vi "S4GUI_002.vi"(7 "Tab ObsEng":enum32{"Obs", "CCD modes", "Eng"}(tab)) -> ()   [LabVIEW 2018] (continued)
            n1189 = call-dynamic "Read TelFocus.lvclass.vi"("error in (no error)"=w302, "S4GUI in"=w303) -> ("error out"=w300:errorcluster, "TelFocus.lvclass"=w301:refnum<class "TelFocus.lvclass">)  [unwired: 7 in, 1 out]
            n1190 = Select(t="STOP", s=w320, f="INIT") -> (s? t:f=w319:string)
            n1191 = call-dynamic "Read focus #stepsdone.vi"("error in (no error)"=w300, "TelFocus in"=w301) -> ("focus #stepsdone"=→"steps done":u32)  [unwired: 7 in, 2 out]
            n1192 = property on="Init mode" class="Bool"(error in=w302, "Blinking"=w320, "Caption.Visible"=w320, "BoolText.Text"=w319) -> (error out=w321:errorcluster)  [unwired: 1 in, 1 out]
            n1193 = call-dynamic "Read cyclesDone.vi"("error in (no error)"=w321, "S4GUI in"=w303) -> ("error out"=w313:errorcluster, "cyclesDone"=w305:u32, "S4GUI out"=w315:refnum<class "S4GUI.lvclass">)  [unwired: 7 in]
            "#Cycles Done" <- w305
            n1194 = call-dynamic "Read cycles wprot.vi"("error in (no error)"=w313, "S4GUI in"=w315) -> ("cycles wprot"=→"Cycles Counter":u32)  [unwired: 7 in, 2 out]
            n1195 = Number To Decimal String(number=w305) -> (decimal integer string=w306:string)  [unwired: 1 in]
            n1196 = Concatenate Strings("#Cycles Done ", w306) -> (w304:string)
            n1197 = property on="#Cycles Done" class="Slide (strict)"("Caption.Text"=w304) -> ()  [unwired: 2 in, 2 out]
            n1198 = call "Read Instrument.lvclass.vi"("error in (no error)"=w313, "S4ACS_GUI in"=w315) -> ("error out"=w330:errorcluster, "Instrument.lvclass"=w328:refnum<class "Instrument.lvclass">, "S4ACS_GUI out"=w331:refnum<class "S4GUI.lvclass">)  [unwired: 7 in]
            n1199 = call-dynamic "Write mode.vi"("error in (no error)"=w330, "mode"=w316, "Instrument in"=w328) -> ("error out"=w329:errorcluster, "Instrument out"=w327:refnum<class "Instrument.lvclass">)  [unwired: 7 in]
            n1200 = call "Write Instrument.lvclass.vi"("error in (no error)"=w329, "Instrument.lvclass"=w327, "S4ACS_GUI in"=w331) -> ("error out"=w311:errorcluster, "S4ACS_GUI out"=w312:refnum<class "S4GUI.lvclass">)  [unwired: 7 in]
            n1201 = call-dynamic "Read Error Msg.vi"("error in (no error)"=w311, "S4GUI in"=w312) -> ("error out"=w308:errorcluster, "Error Msg"=w290:string, "S4GUI out"=w295:refnum<class "S4GUI.lvclass">)  [unwired: 7 in]
            "Last Error" <- w290
            n1202 = Match Pattern(string=w290, regular expression=w309) -> (match substring=w310:string)  [unwired: 1 in, 3 out]
            n1203 = Equal?(x=w310, y=w309) -> (x = y?=w289:bool)
            n1204 = Match Pattern(string=w290, regular expression=w291) -> (match substring=w292:string)  [unwired: 1 in, 3 out]
            n1205 = Equal?(x=w292, y=w291) -> (x = y?=w288:bool)
            n1206 = Or(x=w289, y=w288) -> (x .or. y?=w287:bool)
            n1207 = property on="Last Error" class="Str"(error in=w308, "Blinking"=w287) -> (error out=w293:errorcluster)  [unwired: 1 in, 1 out]
            n1208 = call "Read Instrument.lvclass.vi"("error in (no error)"=w293, "S4ACS_GUI in"=w295) -> ("error out"=w297:errorcluster, "Instrument.lvclass"=w296:refnum<class "Instrument.lvclass">, "S4ACS_GUI out"=w285:refnum<class "S4GUI.lvclass">)  [unwired: 7 in]
            n1209 = call-dynamic "Read mode.vi"("error in (no error)"=w297, "Instrument in"=w296) -> ("error out"=w286:errorcluster, "mode"=w298:bool)  [unwired: 7 in, 1 out]
            n1210 = while {
              tunnel: w298 -> [w341]
              shift-right: [w337] -> _
              shift-left: _ -> [w340]
              shift-right: [w338] -> _
              shift-left: _ -> [w339]
              stop <- TRUE stop-if-true
              n1211 = case shown="False" w341 {
                tunnel: w340 -> [w343 w362]
                tunnel: [w344 w361] -> w337
                tunnel: w339 -> [w346 w360]
                tunnel: [w345 w359] -> w338
                frame True {
                  # "polarimetria"
                  n1212 = case shown="False" w346 {
                    selector: w346 -> [w356 w358]
                    tunnel: [w355 w358] -> w345
                    tunnel: [FALSE FALSE] -> w344
                    tunnel: w343 -> [_ _]
                    frame False {
                      w353 = 11
                      w350 = 80
                      w349 = 12900
                      # "Valor médio\ndo curso do foco."
                      n1213 = local write "Start focus"(w349) -> ()
                      n1214 = local write "Step focus"(w350) -> ()
                      n1215 = local write "#steps"(w353) -> ()
                      n1216 = Quotient & Remainder(x=w353, y=2) -> (floor(x/y)=w351:i32)  [unwired: 1 out]
                      n1217 = Multiply(x=w350, y=w351) -> (x*y=w348:i32)
                      n1218 = Add(x=w349, y=w348) -> (x+y=w347:i32)
                      n1219 = local write "Target focus 2"(w347) -> ()
                      n1220 = local write "Target focus"(w347) -> ()
                      n1221 = Not(x=w356) -> (.not. x?=w355:bool)
                    }
                    frame True {
                    }
                  }
                }
                frame False {
                  # "fotometria"
                  n1222 = case shown="False" w362 {
                    selector: w362 -> [w371 w374]
                    tunnel: [w370 w374] -> w361
                    tunnel: w360 -> [_ _]
                    tunnel: [FALSE FALSE] -> w359
                    frame False {
                      w366 = 11
                      w365 = 100
                      w364 = 13400
                      # "Valor médio\ndo curso do foco."
                      n1223 = local write "Start focus"(w364) -> ()
                      n1224 = local write "Step focus"(w365) -> ()
                      n1225 = local write "#steps"(w366) -> ()
                      n1226 = Quotient & Remainder(x=w366, y=2) -> (floor(x/y)=w368:i32)  [unwired: 1 out]
                      n1227 = Multiply(x=w365, y=w368) -> (x*y=w367:i32)
                      n1228 = Add(x=w364, y=w367) -> (x+y=w363:i32)
                      n1229 = local write "Target focus"(w363) -> ()
                      n1230 = local write "Target focus 2"(w363) -> ()
                      n1231 = Not(x=w371) -> (.not. x?=w370:bool)
                    }
                    frame True {
                    }
                  }
                }
              }
            }
            n1232 = call-dynamic "Read exit.vi"("error in (no error)"=w286, "S4GUI in"=w285) -> ("error out"=w284:errorcluster, "exit"=w283:bool, "S4GUI out"=w282:refnum<class "S4GUI.lvclass">)  [unwired: 7 in]
          }
        }
      }
      event "Lambda Selector": Mouse Down? {
        n1233 = event-data() -> ()  [unwired: 1 in, 7 out]
        n1234 = First Call?() -> (First Call?: T/F=w1982:bool)
        n1235 = case shown="True" w1982 {
          tunnel: w1984 -> [w1986 w1988]
          tunnel: [w1986 w1987] -> w1983
          frame False {
          }
          frame True {
            w1990 = u16 0 items=["OFF", "Lambda/2", "Lambda/4"] ("Lambda Selector")
            n1236 = property on="Lambda Selector" class="Ring (strict)"(error in=w1988, "Value"=w1990) -> (error out=w1991:errorcluster)  [unwired: 1 in, 1 out]
            n1237 = property on="Lambda Selector" class="Ring (strict)"(error in=w1991, "RingText.Text"="OFF" ("Boolean Text.Text")) -> (error out=w1987:errorcluster)  [unwired: 1 in, 1 out]
          }
        }
        n1238 = event-data() -> ()  [unwired: 2 in, 1 out]
      }
      event "object suffix": Key Down; "object suffix": Key Repeat {
        n1239 = event-data() -> ("Char"=w1992:i16)  [unwired: 1 in]
        "charKeyboardInteger" <- w1992
        n1240 = call-dynamic "Write charSuffix.vi"("error in (no error)"=w1995, "charSuffix"=w1992, "S4GUI in"=w1996) -> ("error out"=w1993:errorcluster, "S4GUI out"=w1994:refnum<class "S4GUI.lvclass">)  [unwired: 7 in]
      }
      event "dflat suffix": Key Down; "dflat suffix": Key Repeat {
        n1241 = event-data() -> ("Char"=w1999:i16)  [unwired: 1 in]
        n1242 = call-dynamic "Write charSuffix.vi"("error in (no error)"=w2000, "charSuffix"=w1999, "S4GUI in"=w2001) -> ("error out"=w1997:errorcluster, "S4GUI out"=w1998:refnum<class "S4GUI.lvclass">)  [unwired: 7 in]
      }
      event "sflat suffix": Key Down; "sflat suffix": Key Repeat {
        n1243 = event-data() -> ("Char"=w2004:i16)  [unwired: 1 in]
        n1244 = call-dynamic "Write charSuffix.vi"("error in (no error)"=w2005, "charSuffix"=w2004, "S4GUI in"=w2006) -> ("error out"=w2002:errorcluster, "S4GUI out"=w2003:refnum<class "S4GUI.lvclass">)  [unwired: 7 in]
      }
      event "dark suffix": Key Down; "dark suffix": Key Repeat {
        n1245 = event-data() -> ("Char"=w2009:i16)  [unwired: 1 in]
        n1246 = call-dynamic "Write charSuffix.vi"("error in (no error)"=w2010, "charSuffix"=w2009, "S4GUI in"=w2011) -> ("error out"=w2007:errorcluster, "S4GUI out"=w2008:refnum<class "S4GUI.lvclass">)  [unwired: 7 in]
      }
      event "zero suffix": Key Down; "zero suffix": Key Repeat {
        n1247 = event-data() -> ("Char"=w2014:i16)  [unwired: 1 in]
        n1248 = call-dynamic "Write charSuffix.vi"("error in (no error)"=w2015, "charSuffix"=w2014, "S4GUI in"=w2016) -> ("error out"=w2012:errorcluster, "S4GUI out"=w2013:refnum<class "S4GUI.lvclass">)  [unwired: 7 in]
      }
      event "focus suffix": Key Down; "focus suffix": Key Repeat {
        n1249 = event-data() -> ("Char"=w2019:i16)  [unwired: 1 in]
        n1250 = call-dynamic "Write charSuffix.vi"("error in (no error)"=w2020, "charSuffix"=w2019, "S4GUI in"=w2021) -> ("error out"=w2017:errorcluster, "S4GUI out"=w2018:refnum<class "S4GUI.lvclass">)  [unwired: 7 in]
      }
      event "Set CCD mode": Value Change {
        w2084 = i16 1 items=["Cooler OFF", "Cooler ON"] ("Cooler ON/OFF")
        w2098 = i16 1 items=["Cooler OFF", "Cooler ON"] ("Cooler ON/OFF")
        w2114 = i16 1 items=["Cooler OFF", "Cooler ON"] ("Cooler ON/OFF")
        w2134 = i16 1 items=["Cooler OFF", "Cooler ON"] ("Cooler ON/OFF")
        # "Sinaliza que houve requisição de SET CCD mode"
        n1251 = event-data() -> ()  [unwired: 1 in, 6 out]
        n1252 = call-dynamic "Write User Event.vi"("error in (no error)"=w2292, "User Event"="SET CCD mode ", "S4GUI in"=w2291) -> ("error out"=w2079:errorcluster, "S4GUI out"=w2078:refnum<class "S4GUI.lvclass">)  [unwired: 7 in]
        n1253 = call-dynamic "Write SET request.vi"("error in (no error)"=w2079, "SET request"=TRUE, "S4GUI in"=w2078) -> ("error out"=w2076:errorcluster, "S4GUI out"=w2077:refnum<class "S4GUI.lvclass">)  [unwired: 7 in]
        n1254 = call-dynamic "Read CCD mode.vi"("error in (no error)"=w2076, "S4GUI in"=w2077) -> ("error out"=w2289:errorcluster, "CCD mode"=w2290:T30, "S4GUI out"=w2288:refnum<class "S4GUI.lvclass">)  [unwired: 7 in]
        n1255 = Bundle By Name(cluster=w2290, "FTM"="Frame Transfer", "AQM"="AQM", "SZM"="SZM", "EM gain"="EM Gain") -> (w2287:T30)
        n1256 = call-dynamic "Write CCD mode.vi"("error in (no error)"=w2289, "CCD mode"=w2287, "S4GUI in"=w2288) -> ("error out"=w2145:errorcluster, "S4GUI out"=w2146:refnum<class "S4GUI.lvclass">)  [unwired: 7 in]
        n1257 = call-dynamic "LoadCCDmode.vi"("error in (no error)"=w2145, "S4GUI in"=w2146) -> ("error out"=w2144:errorcluster, "S4GUI out"=w2143:refnum<class "S4GUI.lvclass">)  [unwired: 8 in]
        n1258 = call-dynamic "Read Parameters CCD modes.vi"("error in (no error)"=w2144, "S4GUI in"=w2143) -> ("error out"=w2142:errorcluster, "Parameters CCD modes"=w2147:T5, "S4GUI out"=w2141:refnum<class "S4GUI.lvclass">)  [unwired: 7 in]
        n1259 = Unbundle By Name(w2147) -> ("CCD \nEM Mode"=w2279:u8, "Readout\nRate"=w2139:u8)
        n1260 = case shown="0, Default" w2279 {
          tunnel: [string[] ["30 MHz", "20 MHz", "10 MHz", "1 MHz"] ("Strings []") string[] ["1 MHz", "0.1 MHz"] ("Strings []")] -> w2280
          frame 0, Default {
          }
          frame 1 {
          }
        }
        n1261 = flat-sequence {
          tunnel: w2280 -> [w2426]
          tunnel: w2279 -> [w2427]
          tunnel: [w2427] -> w2281
          tunnel: w2147 -> [w2433]
          tunnel: [w2432] -> w2140
          tunnel: w2281 -> [w2430]
          tunnel: w2148 -> [w2431]
          tunnel: w2139 -> [w2428]
          frame #0 {
            n1262 = property on="Readout\nRate" class="Ring (strict)"("Strings []"=w2426) -> ()  [unwired: 2 in, 2 out]
            n1263 = property on="Readout\nRate" class="Ring (strict)"("Strings []"=w2426) -> ()  [unwired: 2 in, 2 out]
            n1264 = property on="Readout Rate 2" class="Ring (strict)"("Strings []"=w2426) -> ()  [unwired: 2 in, 2 out]
            n1265 = property on="Readout Rate" class="Ring (strict)"("Strings []"=w2426) -> ()  [unwired: 2 in, 2 out]
            n1266 = property on="Readout Rate 3" class="Ring (strict)"("Strings []"=w2426) -> ()  [unwired: 2 in, 2 out]
            n1267 = property on="Readout Rate 4" class="Ring (strict)"("Strings []"=w2426) -> ()  [unwired: 2 in, 2 out]
          }
          frame #1 {
            n1268 = Bundle By Name(cluster=w2433, "Readout\nRate"=w2428, "CCD \nEM Mode"=w2430) -> (w2432:T5)
            n1269 = disable-structure shown="Enabled" {
              disable-tunnel: w2431 -> [w2437 w2438]
              disable-tunnel: w2430 -> [w2436 _]
              disable-tunnel: [w2435 w2438] -> w2429
              disable-tunnel: w2428 -> [w2434 _]
              frame Disabled {
                n1270 = Bundle By Name(cluster=w2437, "Parameters.Readout\nRate"=w2434, "Parameters.CCD \nEM Mode"=w2436) -> (w2435:T8)
              }
              frame Enabled {
              }
            }
            n1271 = local write "Input Cluster"(w2429) -> ()
          }
        }
        n1272 = call-dynamic "Read InfoCCDmode.vi"("error in (no error)"=w2142, "S4GUI in"=w2141) -> ("error out"=w2282:errorcluster, "InfoCCDmode"=w2074:T2, "S4GUI out"=w2283:refnum<class "S4GUI.lvclass">)  [unwired: 7 in]
        "InfoCCDmode" <- w2074
        n1273 = Unbundle By Name(w2074) -> ("MinExpTime"=w2022:dbl)
        n1274 = call-dynamic "Read Parameters CCD modes.vi"("error in (no error)"=w2282, "S4GUI in"=w2283) -> ("error out"=w2276:errorcluster, "Parameters CCD modes"=→"Parameters CCD modes":T5, "S4GUI out"=w2277:refnum<class "S4GUI.lvclass">)  [unwired: 7 in]
        n1275 = local read "Input Cluster"() -> (w2148:T8)
        n1276 = call-dynamic "Write Parameters CCD modes.vi"("error in (no error)"=w2276, "Parameters CCD modes"=w2140, "S4GUI in"=w2277) -> ("error out"=w2255:errorcluster, "S4GUI out"=w2229:refnum<class "S4GUI.lvclass">)  [unwired: 7 in]
        n1277 = Unbundle By Name(w2140) -> ("Frame\nTransfer"=w2183:bool, "Pre-amplification\nGain"=w2182:u8, "Readout\nRate"=w2181:u8, "CCD \nEM Mode"=w2180:u8, "CCD\nEM Gain"=w2179:u16, "Image \nInitial Line"=w2178:u16, "Image\nInitial Column"=w2177:u16, "Image\nFinal Line"=w2166:u16, "Image\nFInal Column"=w2176:u16, "Vertical\nBinning"=w2175:u16, "Horizontal\nBinning"=w2174:u16)
        n1278 = call-dynamic "Read AcquisitionA.vi"("error in (no error)"=w2255, "S4ACS_GUI in"=w2229) -> ("error out"=w2164:errorcluster, "Acquisition.lvclass"=w2165:refnum<class "Acquisition.lvclass">, "S4ACS_GUI out"=w2275:refnum<class "S4GUI.lvclass">)  [unwired: 7 in]
        n1279 = call-dynamic "Read enabled.vi"("error in (no error)"=w2164, "Server in"=w2165) -> ("error out"=w2163:errorcluster, "enabled"=w2161:bool, "Server out"=w2162:refnum<class "Acquisition.lvclass">)  [unwired: 7 in]
        n1280 = call-dynamic "Read Channel.vi"("error in (no error)"=w2163, "Acquisition in"=w2162) -> ("error out"=w2272:errorcluster, "Channel.lvclass"=w2273:refnum<class "Channel.lvclass">, "Acquisition out"=w2274:refnum<class "Acquisition.lvclass">)  [unwired: 7 in]
        n1281 = call-dynamic "Read Interface.vi"("error in (no error)"=w2272, "Channel in"=w2273) -> ("error out"=w2258:errorcluster, "Interface.lvclass"=w2259:refnum<class "Interface.lvclass">, "Channel out"=w2253:refnum<class "Channel.lvclass">)  [unwired: 7 in]
        n1282 = call-dynamic "Write PREV_FT.vi"("error in (no error)"=w2258, "PREV_FT"=w2183, "Interface in"=w2259) -> ("error out"=w2137:errorcluster, "Interface out"=w2136:refnum<class "Interface.lvclass">)  [unwired: 7 in]
        n1283 = call-dynamic "Write Cooler ON_OFF.vi"("error in (no error)"=w2137, "Cooler ON/OFF"=w2134, "Interface in"=w2136) -> ("error out"=w2135:errorcluster, "Interface out"=w2133:refnum<class "Interface.lvclass">)  [unwired: 7 in]
        n1284 = call-dynamic "Read target cluster.vi"("error in (no error)"=w2135, "Channel in"=w2253) -> ("error out"=w2251:errorcluster, "target cluster"=w2250:T31, "Channel out"=w2252:refnum<class "Channel.lvclass">)  [unwired: 7 in]
        n1285 = Bundle By Name(cluster=w2250, "FRAME_TRANSFER"=w2183, "PREAMP"=w2182, "READOUT_RATE"=w2181, "EM_MODE"=w2180, "EM_GAIN"=w2179, "INITIAL_LINE"=w2178, "INITIAL_COLUMN"=w2177, "FINAL_LINE"=w2166, "FINAL_COLUMN"=w2176, "VBIN"=w2175, "HBIN"=w2174) -> (w2130:T31)
        n1286 = call-dynamic "Write target cluster.vi"("error in (no error)"=w2251, "target cluster"=w2130, "Channel in"=w2252) -> ("error out"=w2131:errorcluster, "Channel out"=w2257:refnum<class "Channel.lvclass">)  [unwired: 7 in]
        n1287 = call-dynamic "Set CCD_Config.vi"("error in (no error)"=w2131, "input cluster"=w2130, "Interface in"=w2133) -> ("error out"=w2120:errorcluster, "Interface out"=w2132:refnum<class "Interface.lvclass">)  [unwired: 7 in]
        n1288 = Flatten To String(anything=w2130, error in (no error)=w2131) -> (data string=w2267:string)  [unwired: 2 in, 2 out]
        n1289 = call "Write flatted cluster.vi"("error in (no error)"=w2120, "flatted cluster"=w2267, "Interface in"=w2132) -> ("error out"=w2069:errorcluster, "Interface out"=w2070:refnum<class "Interface.lvclass">)  [unwired: 7 in]
        n1290 = call "Read Exposure Time.vi"("error in (no error)"=w2069, "Interface in"=w2070) -> ("error out"=w2067:errorcluster, "Exposure Time"=w2072:dbl, "Interface out"=w2068:refnum<class "Interface.lvclass">)  [unwired: 7 in]
        n1291 = Greater Or Equal?(x=w2072, y=w2022) -> (x >= y?=w2073:bool)
        n1292 = Select(t=w2072, s=w2073, f=w2022) -> (s? t:f=w2071:dbl)
        n1293 = local write "Exptime ch1"(w2071) -> ()
        n1294 = call "Write Exposure Time.vi"("error in (no error)"=w2067, "Exposure Time"=w2071, "Interface in"=w2068) -> ("error out"=w2066:errorcluster, "Interface out"=w2065:refnum<class "Interface.lvclass">)  [unwired: 7 in]
        n1295 = call-dynamic "Write Interface.vi"("error in (no error)"=w2066, "Interface.lvclass"=w2065, "Channel in"=w2257) -> ("error out"=w2263:errorcluster, "Channel out"=w2265:refnum<class "Channel.lvclass">)  [unwired: 7 in]
        n1296 = call "Write section_name.vi"("error in (no error)"=w2263, "section_name"="CCD_ACS1", "Channel in"=w2265) -> ("error out"=w2262:errorcluster, "Channel out"=w2264:refnum<class "Channel.lvclass">)  [unwired: 7 in]
        n1297 = call-dynamic "save config.vi"("error in (no error)"=w2262, "file config"="lastsaved.cfg", "Channel in"=w2264) -> ("error out"=w2128:errorcluster, "Channel out"=w2129:refnum<class "Channel.lvclass">)  [unwired: 7 in]
        n1298 = call-dynamic "ValidateConfig.vi"("error in (no error)"=w2128, "Channel in"=w2129) -> ("error out"=w2126:errorcluster, "Channel out"=w2127:refnum<class "Channel.lvclass">)  [unwired: 7 in, 1 out]
        n1299 = call-dynamic "Save Temp.vi"("error in (no error)"=w2126, "temp file"="lasttemp.cfg" ("file config"), "Channel in"=w2127) -> ("error out"=w2125:errorcluster, "Channel out"=w2124:refnum<class "Channel.lvclass">)  [unwired: 7 in]
        n1300 = case shown="True" w2161 {
          tunnel: [w2394 w2419] -> w2271
          tunnel: [w2393 w2418] -> w2270
          tunnel: w2124 -> [w2394 w2417]
          tunnel: w2125 -> [w2393 w2416]
          frame False {
          }
          frame True {
            # "Esvazia\na fila."
            n1301 = call-dynamic "Read State Machine.vi"("error in (no error)"=w2416, "Device in"=w2417) -> ("error out"=w2410:errorcluster, "State Machine.lvclass"=w2413:refnum<class "State Machine.lvclass">, "Device out"=w2423:refnum<class "Channel.lvclass">)  [unwired: 7 in]
            n1302 = call-dynamic "Read ref StatesQueue.vi"("error in (no error)"=w2410, "State Machine in"=w2413) -> ("error out"=w2401:errorcluster, "ref StatesQueue"=w2403:refnum<queue>, "State Machine out"=w2412:refnum<class "State Machine.lvclass">)  [unwired: 7 in]
            n1303 = Flush Queue(queue=w2403, error in (no error)=w2401) -> (queue out=w2402:refnum<queue>, error out=w2400:errorcluster)  [unwired: 1 out]
            n1304 = Enqueue Element(queue=w2402, element=u32 60 ("State"), error in (no error)=w2400) -> (queue out=w2415:refnum<queue>, error out=w2409:errorcluster)  [unwired: 1 in, 1 out]
            n1305 = Enqueue Element(queue=w2415, element=u32 45 ("State"), error in (no error)=w2409) -> (queue out=w2414:refnum<queue>, error out=w2408:errorcluster)  [unwired: 1 in, 1 out]
            n1306 = Enqueue Element(queue=w2414, element=u32 35 ("State"), error in (no error)=w2408) -> (queue out=w2398:refnum<queue>, error out=w2397:errorcluster)  [unwired: 1 in, 1 out]
            n1307 = Enqueue Element(queue=w2398, element=u32 37 ("State"), error in (no error)=w2397) -> (queue out=w2395:refnum<queue>, error out=w2396:errorcluster)  [unwired: 1 in, 1 out]
            n1308 = call-dynamic "Write ref StatesQueue.vi"("error in (no error)"=w2396, "ref StatesQueue"=w2395, "State Machine in"=w2412) -> ("error out"=w2404:errorcluster, "State Machine out"=w2411:refnum<class "State Machine.lvclass">)  [unwired: 7 in]
            n1309 = disable-structure shown="Enabled" {
              disable-tunnel: [0 ("State") 45] -> w2420
              frame Enabled {
                # "Vai pra 0 para que\nos estados da fila \nsejam retirados."
              }
              frame Disabled {
                # "Verifica Texp\nantes de tudo."
              }
            }
            n1310 = call-dynamic "Write State.vi"("error in (no error)"=w2404, "State"=w2420, "State Machine in"=w2411) -> ("error out"=w2421:errorcluster, "State Machine out"=w2422:refnum<class "State Machine.lvclass">)  [unwired: 7 in]
            n1311 = call-dynamic "Write State Machine.vi"("error in (no error)"=w2421, "State Machine.lvclass"=w2422, "Device in"=w2423) -> ("error out"=w2418:errorcluster, "Device out"=w2419:refnum<class "Channel.lvclass">)  [unwired: 7 in]
          }
        }
        n1312 = call-dynamic "Write Channel.vi"("error in (no error)"=w2270, "Channel.lvclass"=w2271, "Acquisition in"=w2274) -> ("error out"=w2269:errorcluster, "Acquisition out"=w2268:refnum<class "Acquisition.lvclass">)  [unwired: 7 in]
        n1313 = call-dynamic "Write AcquisitionA.vi"("error in (no error)"=w2269, "Acquisition.lvclass"=w2268, "S4ACS_GUI in"=w2275) -> ("error out"=w2171:errorcluster, "S4ACS_GUI out"=w2228:refnum<class "S4GUI.lvclass">)  [unwired: 7 in]
        n1314 = call "Read AcquisitionB.vi"("error in (no error)"=errorcluster {"status"=FALSE, "code"=0, "source"=""}, "S4ACS_GUI in"=w2228) -> ("error out"=w2157:errorcluster, "Acquisition.lvclass"=w2160:refnum<class "Acquisition.lvclass">, "S4ACS_GUI out"=w2249:refnum<class "S4GUI.lvclass">)  [unwired: 7 in]
        n1315 = call-dynamic "Read enabled.vi"("error in (no error)"=w2157, "Server in"=w2160) -> ("error out"=w2158:errorcluster, "enabled"=w2050:bool, "Server out"=w2159:refnum<class "Acquisition.lvclass">)  [unwired: 7 in]
        n1316 = call-dynamic "Read Channel.vi"("error in (no error)"=w2158, "Acquisition in"=w2159) -> ("error out"=w2246:errorcluster, "Channel.lvclass"=w2247:refnum<class "Channel.lvclass">, "Acquisition out"=w2248:refnum<class "Acquisition.lvclass">)  [unwired: 7 in]
        n1317 = call-dynamic "Read Interface.vi"("error in (no error)"=w2246, "Channel in"=w2247) -> ("error out"=w2235:errorcluster, "Interface.lvclass"=w2236:refnum<class "Interface.lvclass">, "Channel out"=w2233:refnum<class "Channel.lvclass">)  [unwired: 7 in]
        n1318 = call-dynamic "Write PREV_FT.vi"("error in (no error)"=w2235, "PREV_FT"=w2183, "Interface in"=w2236) -> ("error out"=w2115:errorcluster, "Interface out"=w2117:refnum<class "Interface.lvclass">)  [unwired: 7 in]
        n1319 = call-dynamic "Write Cooler ON_OFF.vi"("error in (no error)"=w2115, "Cooler ON/OFF"=w2114, "Interface in"=w2117) -> ("error out"=w2113:errorcluster, "Interface out"=w2116:refnum<class "Interface.lvclass">)  [unwired: 7 in]
        n1320 = call-dynamic "Read target cluster.vi"("error in (no error)"=w2113, "Channel in"=w2233) -> ("error out"=w2231:errorcluster, "target cluster"=w2230:T31, "Channel out"=w2232:refnum<class "Channel.lvclass">)  [unwired: 7 in]
        n1321 = Bundle By Name(cluster=w2230, "FRAME_TRANSFER"=w2183, "PREAMP"=w2182, "READOUT_RATE"=w2181, "EM_MODE"=w2180, "EM_GAIN"=w2179, "INITIAL_LINE"=w2178, "INITIAL_COLUMN"=w2177, "FINAL_LINE"=w2166, "FINAL_COLUMN"=w2176, "VBIN"=w2175, "HBIN"=w2174) -> (w2118:T31)
        n1322 = call-dynamic "Write target cluster.vi"("error in (no error)"=w2231, "target cluster"=w2118, "Channel in"=w2232) -> ("error out"=w2121:errorcluster, "Channel out"=w2234:refnum<class "Channel.lvclass">)  [unwired: 7 in]
        n1323 = call-dynamic "Set CCD_Config.vi"("error in (no error)"=w2121, "input cluster"=w2118, "Interface in"=w2116) -> ("error out"=w2119:errorcluster, "Interface out"=w2122:refnum<class "Interface.lvclass">)  [unwired: 7 in]
        n1324 = Flatten To String(anything=w2118, error in (no error)=w2121) -> (data string=w2243:string)  [unwired: 2 in, 2 out]
        n1325 = call "Write flatted cluster.vi"("error in (no error)"=w2119, "flatted cluster"=w2243, "Interface in"=w2122) -> ("error out"=w2043:errorcluster, "Interface out"=w2044:refnum<class "Interface.lvclass">)  [unwired: 7 in]
        n1326 = call "Read Exposure Time.vi"("error in (no error)"=w2043, "Interface in"=w2044) -> ("error out"=w2064:errorcluster, "Exposure Time"=w2045:dbl, "Interface out"=w2063:refnum<class "Interface.lvclass">)  [unwired: 7 in]
        n1327 = Greater Or Equal?(x=w2045, y=w2022) -> (x >= y?=w2061:bool)
        n1328 = Select(t=w2045, s=w2061, f=w2022) -> (s? t:f=w2062:dbl)
        n1329 = local write "Exptime ch2"(w2062) -> ()
        n1330 = call "Write Exposure Time.vi"("error in (no error)"=w2064, "Exposure Time"=w2062, "Interface in"=w2063) -> ("error out"=w2042:errorcluster, "Interface out"=w2041:refnum<class "Interface.lvclass">)  [unwired: 7 in]
        n1331 = call-dynamic "Write Interface.vi"("error in (no error)"=w2042, "Interface.lvclass"=w2041, "Channel in"=w2234) -> ("error out"=w2239:errorcluster, "Channel out"=w2241:refnum<class "Channel.lvclass">)  [unwired: 7 in]
        n1332 = call "Write section_name.vi"("error in (no error)"=w2239, "section_name"="CCD_ACS2", "Channel in"=w2241) -> ("error out"=w2238:errorcluster, "Channel out"=w2240:refnum<class "Channel.lvclass">)  [unwired: 7 in]
        n1333 = call-dynamic "save config.vi"("error in (no error)"=w2238, "file config"="lastsaved.cfg", "Channel in"=w2240) -> ("error out"=w2108:errorcluster, "Channel out"=w2109:refnum<class "Channel.lvclass">)  [unwired: 7 in]
        n1334 = call-dynamic "ValidateConfig.vi"("error in (no error)"=w2108, "Channel in"=w2109) -> ("error out"=w2111:errorcluster, "Channel out"=w2112:refnum<class "Channel.lvclass">)  [unwired: 7 in, 1 out]
        n1335 = call-dynamic "Save Temp.vi"("error in (no error)"=w2111, "temp file"="lasttemp.cfg" ("file config"), "Channel in"=w2112) -> ("error out"=w2048:errorcluster, "Channel out"=w2049:refnum<class "Channel.lvclass">)  [unwired: 7 in]
        n1336 = case shown="True" w2050 {
          tunnel: [w2328 w2353] -> w2047
          tunnel: [w2327 w2352] -> w2046
          tunnel: w2049 -> [w2328 w2351]
          tunnel: w2048 -> [w2327 w2350]
          frame False {
          }
          frame True {
            # "Esvazia\na fila."
            n1337 = call-dynamic "Read State Machine.vi"("error in (no error)"=w2350, "Device in"=w2351) -> ("error out"=w2344:errorcluster, "State Machine.lvclass"=w2347:refnum<class "State Machine.lvclass">, "Device out"=w2357:refnum<class "Channel.lvclass">)  [unwired: 7 in]
            n1338 = call-dynamic "Read ref StatesQueue.vi"("error in (no error)"=w2344, "State Machine in"=w2347) -> ("error out"=w2334:errorcluster, "ref StatesQueue"=w2336:refnum<queue>, "State Machine out"=w2346:refnum<class "State Machine.lvclass">)  [unwired: 7 in]
            n1339 = Flush Queue(queue=w2336, error in (no error)=w2334) -> (queue out=w2335:refnum<queue>, error out=w2333:errorcluster)  [unwired: 1 out]
            n1340 = Enqueue Element(queue=w2335, element=u32 60 ("State"), error in (no error)=w2333) -> (queue out=w2349:refnum<queue>, error out=w2343:errorcluster)  [unwired: 1 in, 1 out]
            n1341 = Enqueue Element(queue=w2349, element=u32 45 ("State"), error in (no error)=w2343) -> (queue out=w2348:refnum<queue>, error out=w2342:errorcluster)  [unwired: 1 in, 1 out]
            n1342 = Enqueue Element(queue=w2348, element=u32 35 ("State"), error in (no error)=w2342) -> (queue out=w2341:refnum<queue>, error out=w2331:errorcluster)  [unwired: 1 in, 1 out]
            n1343 = Enqueue Element(queue=w2341, element=u32 37, error in (no error)=w2331) -> (queue out=w2332:refnum<queue>, error out=w2330:errorcluster)  [unwired: 1 in, 1 out]
            n1344 = call-dynamic "Write ref StatesQueue.vi"("error in (no error)"=w2330, "ref StatesQueue"=w2332, "State Machine in"=w2346) -> ("error out"=w2337:errorcluster, "State Machine out"=w2345:refnum<class "State Machine.lvclass">)  [unwired: 7 in]
            n1345 = disable-structure shown="Enabled" {
              disable-tunnel: [0 ("State") 45] -> w2354
              frame Enabled {
                # "Vai pra 0 para que\nos estados da fila \nsejam retirados."
              }
              frame Disabled {
                # "Verifica Texp\nantes de tudo."
              }
            }
            n1346 = call-dynamic "Write State.vi"("error in (no error)"=w2337, "State"=w2354, "State Machine in"=w2345) -> ("error out"=w2355:errorcluster, "State Machine out"=w2356:refnum<class "State Machine.lvclass">)  [unwired: 7 in]
            n1347 = call-dynamic "Write State Machine.vi"("error in (no error)"=w2355, "State Machine.lvclass"=w2356, "Device in"=w2357) -> ("error out"=w2352:errorcluster, "Device out"=w2353:refnum<class "Channel.lvclass">)  [unwired: 7 in]
          }
        }
        n1348 = call-dynamic "Write Channel.vi"("error in (no error)"=w2046, "Channel.lvclass"=w2047, "Acquisition in"=w2248) -> ("error out"=w2245:errorcluster, "Acquisition out"=w2244:refnum<class "Acquisition.lvclass">)  [unwired: 7 in]
        n1349 = call "Write AcquisitionB.vi"("error in (no error)"=w2245, "Acquisition.lvclass"=w2244, "S4ACS_GUI in"=w2249) -> ("error out"=w2170:errorcluster, "S4ACS_GUI out"=w2205:refnum<class "S4GUI.lvclass">)  [unwired: 7 in]
        n1350 = call-dynamic "Read AcquisitionC.vi"("error in (no error)"=errorcluster {"status"=FALSE, "code"=0, "source"=""}, "S4ACS_GUI in"=w2205) -> ("error out"=w2154:errorcluster, "Acquisition.lvclass"=w2156:refnum<class "Acquisition.lvclass">, "S4ACS_GUI out"=w2226:refnum<class "S4GUI.lvclass">)  [unwired: 7 in]
        n1351 = call-dynamic "Read enabled.vi"("error in (no error)"=w2154, "Server in"=w2156) -> ("error out"=w2153:errorcluster, "enabled"=w2040:bool, "Server out"=w2155:refnum<class "Acquisition.lvclass">)  [unwired: 7 in]
        n1352 = call-dynamic "Read Channel.vi"("error in (no error)"=w2153, "Acquisition in"=w2155) -> ("error out"=w2223:errorcluster, "Channel.lvclass"=w2224:refnum<class "Channel.lvclass">, "Acquisition out"=w2225:refnum<class "Acquisition.lvclass">)  [unwired: 7 in]
        n1353 = call-dynamic "Read Interface.vi"("error in (no error)"=w2223, "Channel in"=w2224) -> ("error out"=w2212:errorcluster, "Interface.lvclass"=w2213:refnum<class "Interface.lvclass">, "Channel out"=w2210:refnum<class "Channel.lvclass">)  [unwired: 7 in]
        n1354 = call-dynamic "Write PREV_FT.vi"("error in (no error)"=w2212, "PREV_FT"=w2183, "Interface in"=w2213) -> ("error out"=w2095:errorcluster, "Interface out"=w2097:refnum<class "Interface.lvclass">)  [unwired: 7 in]
        n1355 = call-dynamic "Write Cooler ON_OFF.vi"("error in (no error)"=w2095, "Cooler ON/OFF"=w2098, "Interface in"=w2097) -> ("error out"=w2094:errorcluster, "Interface out"=w2096:refnum<class "Interface.lvclass">)  [unwired: 7 in]
        n1356 = call-dynamic "Read target cluster.vi"("error in (no error)"=w2094, "Channel in"=w2210) -> ("error out"=w2208:errorcluster, "target cluster"=w2207:T31, "Channel out"=w2209:refnum<class "Channel.lvclass">)  [unwired: 7 in]
        n1357 = Bundle By Name(cluster=w2207, "FRAME_TRANSFER"=w2183, "PREAMP"=w2182, "READOUT_RATE"=w2181, "EM_MODE"=w2180, "EM_GAIN"=w2179, "INITIAL_LINE"=w2178, "INITIAL_COLUMN"=w2177, "FINAL_LINE"=w2166, "FINAL_COLUMN"=w2176, "VBIN"=w2175, "HBIN"=w2174) -> (w2102:T31)
        n1358 = call-dynamic "Write target cluster.vi"("error in (no error)"=w2208, "target cluster"=w2102, "Channel in"=w2209) -> ("error out"=w2101:errorcluster, "Channel out"=w2211:refnum<class "Channel.lvclass">)  [unwired: 7 in]
        n1359 = call-dynamic "Set CCD_Config.vi"("error in (no error)"=w2101, "input cluster"=w2102, "Interface in"=w2096) -> ("error out"=w2100:errorcluster, "Interface out"=w2099:refnum<class "Interface.lvclass">)  [unwired: 7 in]
        n1360 = Flatten To String(anything=w2102, error in (no error)=w2101) -> (data string=w2220:string)  [unwired: 2 in, 2 out]
        n1361 = call "Write flatted cluster.vi"("error in (no error)"=w2100, "flatted cluster"=w2220, "Interface in"=w2099) -> ("error out"=w2034:errorcluster, "Interface out"=w2035:refnum<class "Interface.lvclass">)  [unwired: 7 in]
        n1362 = call "Read Exposure Time.vi"("error in (no error)"=w2034, "Interface in"=w2035) -> ("error out"=w2056:errorcluster, "Exposure Time"=w2059:dbl, "Interface out"=w2057:refnum<class "Interface.lvclass">)  [unwired: 7 in]
        n1363 = Greater Or Equal?(x=w2059, y=w2022) -> (x >= y?=w2060:bool)
        n1364 = Select(t=w2059, s=w2060, f=w2022) -> (s? t:f=w2058:dbl)
        n1365 = local write "Exptime ch3"(w2058) -> ()
        n1366 = call "Write Exposure Time.vi"("error in (no error)"=w2056, "Exposure Time"=w2058, "Interface in"=w2057) -> ("error out"=w2032:errorcluster, "Interface out"=w2033:refnum<class "Interface.lvclass">)  [unwired: 7 in]
        n1367 = call-dynamic "Write Interface.vi"("error in (no error)"=w2032, "Interface.lvclass"=w2033, "Channel in"=w2211) -> ("error out"=w2216:errorcluster, "Channel out"=w2218:refnum<class "Channel.lvclass">)  [unwired: 7 in]
        n1368 = call "Write section_name.vi"("error in (no error)"=w2216, "section_name"="CCD_ACS3", "Channel in"=w2218) -> ("error out"=w2215:errorcluster, "Channel out"=w2217:refnum<class "Channel.lvclass">)  [unwired: 7 in]
        n1369 = call-dynamic "save config.vi"("error in (no error)"=w2215, "file config"="lastsaved.cfg", "Channel in"=w2217) -> ("error out"=w2103:errorcluster, "Channel out"=w2104:refnum<class "Channel.lvclass">)  [unwired: 7 in]
        n1370 = call-dynamic "ValidateConfig.vi"("error in (no error)"=w2103, "Channel in"=w2104) -> ("error out"=w2106:errorcluster, "Channel out"=w2107:refnum<class "Channel.lvclass">)  [unwired: 7 in, 1 out]
        n1371 = call-dynamic "Save Temp.vi"("error in (no error)"=w2106, "temp file"="lasttemp.cfg" ("file config"), "Channel in"=w2107) -> ("error out"=w2038:errorcluster, "Channel out"=w2039:refnum<class "Channel.lvclass">)  [unwired: 7 in]
        n1372 = case shown="True" w2040 {
          tunnel: [w2295 w2320] -> w2037
          tunnel: [w2294 w2319] -> w2036
          tunnel: w2039 -> [w2295 w2318]
          tunnel: w2038 -> [w2294 w2317]
          frame False {
          }
          frame True {
            # "Esvazia\na fila."
            n1373 = call-dynamic "Read State Machine.vi"("error in (no error)"=w2317, "Device in"=w2318) -> ("error out"=w2311:errorcluster, "State Machine.lvclass"=w2314:refnum<class "State Machine.lvclass">, "Device out"=w2324:refnum<class "Channel.lvclass">)  [unwired: 7 in]
            n1374 = call-dynamic "Read ref StatesQueue.vi"("error in (no error)"=w2311, "State Machine in"=w2314) -> ("error out"=w2301:errorcluster, "ref StatesQueue"=w2303:refnum<queue>, "State Machine out"=w2313:refnum<class "State Machine.lvclass">)  [unwired: 7 in]
            n1375 = Flush Queue(queue=w2303, error in (no error)=w2301) -> (queue out=w2302:refnum<queue>, error out=w2300:errorcluster)  [unwired: 1 out]
            n1376 = Enqueue Element(queue=w2302, element=u32 60 ("State"), error in (no error)=w2300) -> (queue out=w2316:refnum<queue>, error out=w2310:errorcluster)  [unwired: 1 in, 1 out]
            n1377 = Enqueue Element(queue=w2316, element=u32 45 ("State"), error in (no error)=w2310) -> (queue out=w2315:refnum<queue>, error out=w2309:errorcluster)  [unwired: 1 in, 1 out]
            n1378 = Enqueue Element(queue=w2315, element=u32 35 ("State"), error in (no error)=w2309) -> (queue out=w2308:refnum<queue>, error out=w2298:errorcluster)  [unwired: 1 in, 1 out]
            n1379 = Enqueue Element(queue=w2308, element=u32 37, error in (no error)=w2298) -> (queue out=w2299:refnum<queue>, error out=w2297:errorcluster)  [unwired: 1 in, 1 out]
            n1380 = call-dynamic "Write ref StatesQueue.vi"("error in (no error)"=w2297, "ref StatesQueue"=w2299, "State Machine in"=w2313) -> ("error out"=w2304:errorcluster, "State Machine out"=w2312:refnum<class "State Machine.lvclass">)  [unwired: 7 in]
            n1381 = disable-structure shown="Enabled" {
              disable-tunnel: [0 ("State") 45] -> w2321
              frame Enabled {
                # "Vai pra 0 para que\nos estados da fila \nsejam retirados."
              }
              frame Disabled {
                # "Verifica Texp\nantes de tudo."
              }
            }
            n1382 = call-dynamic "Write State.vi"("error in (no error)"=w2304, "State"=w2321, "State Machine in"=w2312) -> ("error out"=w2322:errorcluster, "State Machine out"=w2323:refnum<class "State Machine.lvclass">)  [unwired: 7 in]
            n1383 = call-dynamic "Write State Machine.vi"("error in (no error)"=w2322, "State Machine.lvclass"=w2323, "Device in"=w2324) -> ("error out"=w2319:errorcluster, "Device out"=w2320:refnum<class "Channel.lvclass">)  [unwired: 7 in]
          }
        }
        n1384 = call-dynamic "Write Channel.vi"("error in (no error)"=w2036, "Channel.lvclass"=w2037, "Acquisition in"=w2225) -> ("error out"=w2222:errorcluster, "Acquisition out"=w2221:refnum<class "Acquisition.lvclass">)  [unwired: 7 in]
        n1385 = call-dynamic "Write AcquisitionC.vi"("error in (no error)"=w2222, "Acquisition.lvclass"=w2221, "S4ACS_GUI in"=w2226) -> ("error out"=w2169:errorcluster, "S4ACS_GUI out"=w2173:refnum<class "S4GUI.lvclass">)  [unwired: 7 in]
        n1386 = call-dynamic "Read AcquisitionD.vi"("error in (no error)"=errorcluster {"status"=FALSE, "code"=0, "source"=""}, "S4ACS_GUI in"=w2173) -> ("error out"=w2150:errorcluster, "Acquisition.lvclass"=w2152:refnum<class "Acquisition.lvclass">, "S4ACS_GUI out"=w2204:refnum<class "S4GUI.lvclass">)  [unwired: 7 in]
        n1387 = call-dynamic "Read enabled.vi"("error in (no error)"=w2150, "Server in"=w2152) -> ("error out"=w2149:errorcluster, "enabled"=w2031:bool, "Server out"=w2151:refnum<class "Acquisition.lvclass">)  [unwired: 7 in]
        n1388 = call-dynamic "Read Channel.vi"("error in (no error)"=w2149, "Acquisition in"=w2151) -> ("error out"=w2201:errorcluster, "Channel.lvclass"=w2202:refnum<class "Channel.lvclass">, "Acquisition out"=w2203:refnum<class "Acquisition.lvclass">)  [unwired: 7 in]
        n1389 = call-dynamic "Read Interface.vi"("error in (no error)"=w2201, "Channel in"=w2202) -> ("error out"=w2190:errorcluster, "Interface.lvclass"=w2191:refnum<class "Interface.lvclass">, "Channel out"=w2188:refnum<class "Channel.lvclass">)  [unwired: 7 in]
        n1390 = call-dynamic "Write PREV_FT.vi"("error in (no error)"=w2190, "PREV_FT"=w2183, "Interface in"=w2191) -> ("error out"=w2083:errorcluster, "Interface out"=w2082:refnum<class "Interface.lvclass">)  [unwired: 7 in]
        n1391 = call-dynamic "Write Cooler ON_OFF.vi"("error in (no error)"=w2083, "Cooler ON/OFF"=w2084, "Interface in"=w2082) -> ("error out"=w2080:errorcluster, "Interface out"=w2081:refnum<class "Interface.lvclass">)  [unwired: 7 in]
        n1392 = call-dynamic "Read target cluster.vi"("error in (no error)"=w2080, "Channel in"=w2188) -> ("error out"=w2186:errorcluster, "target cluster"=w2185:T31, "Channel out"=w2187:refnum<class "Channel.lvclass">)  [unwired: 7 in]
        n1393 = Bundle By Name(cluster=w2185, "FRAME_TRANSFER"=w2183, "PREAMP"=w2182, "READOUT_RATE"=w2181, "EM_MODE"=w2180, "EM_GAIN"=w2179, "INITIAL_LINE"=w2178, "INITIAL_COLUMN"=w2177, "FINAL_LINE"=w2166, "FINAL_COLUMN"=w2176, "VBIN"=w2175, "HBIN"=w2174) -> (w2085:T31)
        n1394 = call-dynamic "Write target cluster.vi"("error in (no error)"=w2186, "target cluster"=w2085, "Channel in"=w2187) -> ("error out"=w2086:errorcluster, "Channel out"=w2189:refnum<class "Channel.lvclass">)  [unwired: 7 in]
        n1395 = call-dynamic "Set CCD_Config.vi"("error in (no error)"=w2086, "input cluster"=w2085, "Interface in"=w2081) -> ("error out"=w2087:errorcluster, "Interface out"=w2088:refnum<class "Interface.lvclass">)  [unwired: 7 in]
        n1396 = Flatten To String(anything=w2085, error in (no error)=w2086) -> (data string=w2198:string)  [unwired: 2 in, 2 out]
        n1397 = call "Write flatted cluster.vi"("error in (no error)"=w2087, "flatted cluster"=w2198, "Interface in"=w2088) -> ("error out"=w2025:errorcluster, "Interface out"=w2026:refnum<class "Interface.lvclass">)  [unwired: 7 in]
        n1398 = call "Read Exposure Time.vi"("error in (no error)"=w2025, "Interface in"=w2026) -> ("error out"=w2055:errorcluster, "Exposure Time"=w2052:dbl, "Interface out"=w2054:refnum<class "Interface.lvclass">)  [unwired: 7 in]
        n1399 = Greater Or Equal?(x=w2052, y=w2022) -> (x >= y?=w2051:bool)
        n1400 = Select(t=w2052, s=w2051, f=w2022) -> (s? t:f=w2053:dbl)
        n1401 = local write "Exptime ch4"(w2053) -> ()
        n1402 = call "Write Exposure Time.vi"("error in (no error)"=w2055, "Exposure Time"=w2053, "Interface in"=w2054) -> ("error out"=w2023:errorcluster, "Interface out"=w2024:refnum<class "Interface.lvclass">)  [unwired: 7 in]
        n1403 = call-dynamic "Write Interface.vi"("error in (no error)"=w2023, "Interface.lvclass"=w2024, "Channel in"=w2189) -> ("error out"=w2194:errorcluster, "Channel out"=w2196:refnum<class "Channel.lvclass">)  [unwired: 7 in]
        n1404 = call "Write section_name.vi"("error in (no error)"=w2194, "section_name"="CCD_ACS4", "Channel in"=w2196) -> ("error out"=w2193:errorcluster, "Channel out"=w2195:refnum<class "Channel.lvclass">)  [unwired: 7 in]
        n1405 = call-dynamic "save config.vi"("error in (no error)"=w2193, "file config"="lastsaved.cfg", "Channel in"=w2195) -> ("error out"=w2089:errorcluster, "Channel out"=w2090:refnum<class "Channel.lvclass">)  [unwired: 7 in]
        n1406 = call-dynamic "ValidateConfig.vi"("error in (no error)"=w2089, "Channel in"=w2090) -> ("error out"=w2092:errorcluster, "Channel out"=w2093:refnum<class "Channel.lvclass">)  [unwired: 7 in, 1 out]
        n1407 = call-dynamic "Save Temp.vi"("error in (no error)"=w2092, "temp file"="lasttemp.cfg" ("file config"), "Channel in"=w2093) -> ("error out"=w2028:errorcluster, "Channel out"=w2027:refnum<class "Channel.lvclass">)  [unwired: 7 in]
        n1408 = case shown="True" w2031 {
          tunnel: [w2360 w2386] -> w2030
          tunnel: [w2361 w2385] -> w2029
          tunnel: w2028 -> [w2361 w2384]
          tunnel: w2027 -> [w2360 w2366]
          frame False {
          }
          frame True {
            # "Esvazia\na fila."
            n1409 = call-dynamic "Read State Machine.vi"("error in (no error)"=w2384, "Device in"=w2366) -> ("error out"=w2378:errorcluster, "State Machine.lvclass"=w2381:refnum<class "State Machine.lvclass">, "Device out"=w2390:refnum<class "Channel.lvclass">)  [unwired: 7 in]
            n1410 = call-dynamic "Read ref StatesQueue.vi"("error in (no error)"=w2378, "State Machine in"=w2381) -> ("error out"=w2368:errorcluster, "ref StatesQueue"=w2370:refnum<queue>, "State Machine out"=w2380:refnum<class "State Machine.lvclass">)  [unwired: 7 in]
            n1411 = Flush Queue(queue=w2370, error in (no error)=w2368) -> (queue out=w2369:refnum<queue>, error out=w2367:errorcluster)  [unwired: 1 out]
            n1412 = Enqueue Element(queue=w2369, element=u32 60 ("State"), error in (no error)=w2367) -> (queue out=w2383:refnum<queue>, error out=w2377:errorcluster)  [unwired: 1 in, 1 out]
            n1413 = Enqueue Element(queue=w2383, element=u32 45 ("State"), error in (no error)=w2377) -> (queue out=w2382:refnum<queue>, error out=w2376:errorcluster)  [unwired: 1 in, 1 out]
            n1414 = Enqueue Element(queue=w2382, element=u32 35 ("State"), error in (no error)=w2376) -> (queue out=w2375:refnum<queue>, error out=w2364:errorcluster)  [unwired: 1 in, 1 out]
            n1415 = Enqueue Element(queue=w2375, element=u32 37, error in (no error)=w2364) -> (queue out=w2365:refnum<queue>, error out=w2363:errorcluster)  [unwired: 1 in, 1 out]
            n1416 = call-dynamic "Write ref StatesQueue.vi"("error in (no error)"=w2363, "ref StatesQueue"=w2365, "State Machine in"=w2380) -> ("error out"=w2371:errorcluster, "State Machine out"=w2379:refnum<class "State Machine.lvclass">)  [unwired: 7 in]
            n1417 = disable-structure shown="Enabled" {
              disable-tunnel: [0 ("State") 45] -> w2387
              frame Enabled {
                # "Vai pra 0 para que\nos estados da fila \nsejam retirados."
              }
              frame Disabled {
                # "Verifica Texp\nantes de tudo."
              }
            }
            n1418 = call-dynamic "Write State.vi"("error in (no error)"=w2371, "State"=w2387, "State Machine in"=w2379) -> ("error out"=w2388:errorcluster, "State Machine out"=w2389:refnum<class "State Machine.lvclass">)  [unwired: 7 in]
            n1419 = call-dynamic "Write State Machine.vi"("error in (no error)"=w2388, "State Machine.lvclass"=w2389, "Device in"=w2390) -> ("error out"=w2385:errorcluster, "Device out"=w2386:refnum<class "Channel.lvclass">)  [unwired: 7 in]
          }
        }
        n1420 = call-dynamic "Write Channel.vi"("error in (no error)"=w2029, "Channel.lvclass"=w2030, "Acquisition in"=w2203) -> ("error out"=w2200:errorcluster, "Acquisition out"=w2199:refnum<class "Acquisition.lvclass">)  [unwired: 7 in]
        n1421 = call-dynamic "Write AcquisitionD.vi"("error in (no error)"=w2200, "Acquisition.lvclass"=w2199, "S4ACS_GUI in"=w2204) -> ("error out"=w2168:errorcluster, "S4ACS_GUI out"=w2172:refnum<class "S4GUI.lvclass">)  [unwired: 7 in]
        n1422 = Merge Errors(w2171, w2170, w2169, w2168) -> (w2167:errorcluster)
        n1423 = call "Write cfg file.vi"("error in (no error)"=w2167, "cfg file"="lastsaved.cfg", "S4ACS_GUI in"=w2172) -> ("error out"=w2254:errorcluster, "S4ACS_GUI out"=w2256:refnum<class "S4GUI.lvclass">)  [unwired: 7 in]
      }
      event "Frame Transfer", "AQM", "SZM", "EM Gain": Value Change {
        # "criar  S4GUI:CalcTemp.vi (metodo da classe S4GUI.lvclass)\na mesma lógica do Channel:ValidateConfig.vi usando\no cluster S4GUI:Parameters CCD em vez do cluster Interface:CCD CF.\nIgnore o Texp Min e apenas salve a temperatura em S4GUI:PrevTemp"
        # "Sinaliza que não há requisição de SET CCD mode"
        n1424 = event-data() -> ()  [unwired: 1 in, 6 out]
        n1425 = call-dynamic "Write SET request.vi"("error in (no error)"=w2448, "SET request"=FALSE, "S4GUI in"=w2450) -> ("error out"=w2447:errorcluster, "S4GUI out"=w2449:refnum<class "S4GUI.lvclass">)  [unwired: 7 in]
        n1426 = local read "Frame Transfer"() -> (w2463:enum16{"OFF", "ON"})
        n1427 = local read "EM Gain"() -> (w2452:u16)
        n1428 = local read "AQM"() -> (w2462:T4)
        n1429 = local read "SZM"() -> (w2461:T3)
        n1430 = call-dynamic "Read CCD mode.vi"("error in (no error)"=w2447, "S4GUI in"=w2449) -> ("error out"=w2460:errorcluster, "CCD mode"=w2465:T30, "S4GUI out"=w2466:refnum<class "S4GUI.lvclass">)  [unwired: 7 in]
        n1431 = Bundle By Name(cluster=w2465, "FTM"=w2463, "AQM"=w2462, "SZM"=w2461, "EM gain"=w2452) -> (w2464:T30)
        n1432 = call-dynamic "Write CCD mode.vi"("error in (no error)"=w2460, "CCD mode"=w2464, "S4GUI in"=w2466) -> ("error out"=w2458:errorcluster, "S4GUI out"=w2459:refnum<class "S4GUI.lvclass">)  [unwired: 7 in]
        n1433 = call-dynamic "LoadCCDmode.vi"("error in (no error)"=w2458, "S4GUI in"=w2459) -> ("error out"=w2456:errorcluster, "S4GUI out"=w2457:refnum<class "S4GUI.lvclass">)  [unwired: 8 in]
        n1434 = call-dynamic "Read Parameters CCD modes.vi"("error in (no error)"=w2456, "S4GUI in"=w2457) -> ("error out"=w2453:errorcluster, "Parameters CCD modes"=w2451:T5, "S4GUI out"=w2455:refnum<class "S4GUI.lvclass">)  [unwired: 7 in]
        n1435 = call-dynamic "Read InfoCCDmode.vi"("error in (no error)"=w2453, "S4GUI in"=w2455) -> ("error out"=w2443:errorcluster, "InfoCCDmode"=w2454:T2, "S4GUI out"=w2444:refnum<class "S4GUI.lvclass">)  [unwired: 7 in]
        n1436 = local write "Parameters CCD modes"(w2451) -> ()
        n1437 = local write "InfoCCDmode"(w2454) -> ()
        n1438 = call-dynamic "CalcTemp.vi"("error in (no error)"=w2443, "S4GUI in"=w2444) -> ("error out"=w2442:errorcluster, "S4GUI out"=w2441:refnum<class "S4GUI.lvclass">)  [unwired: 8 in]
        n1439 = call-dynamic "Read Prev Temp.vi"("error in (no error)"=w2442, "S4GUI in"=w2441) -> ("Prev Temp"=→"Preview Temp.":dbl)  [unwired: 7 in, 2 out]
      }
      event "TCS mode": Value Change {
        # "2024-04-04: Não se usa mais o ID para configurar a comunicação..."
        # "simul"
        # "real"
        # "Inicializar nova comunicação, de acordo\n com valor de TCS mode\n\nServer.Write id (T=6 ou F=12)\nTCS.Init"
        # "Parar a comunciação atual\nServer.End"
        n1440 = event-data() -> ("NewVal"=w2469:bool)  [unwired: 1 in, 5 out]
        n1441 = call-dynamic "Read TCS.lvclass.vi"("error in (no error)"=w2479, "S4GUI in"=w2480) -> ("error out"=w2474:errorcluster, "TCS.lvclass"=w2477:refnum<class "TCS.lvclass">, "S4GUI out"=w2478:refnum<class "S4GUI.lvclass">)  [unwired: 7 in]
        n1442 = call-dynamic "End.vi"("error in (no error)"=w2474, "Server in"=w2477) -> ("error out"=w2473:errorcluster, "Server out"=w2476:refnum<class "TCS.lvclass">)  [unwired: 8 in]
        n1443 = Select(t=u32 6, s=w2469, f=u32 12) -> (s? t:f=w2483:u32)
        n1444 = call-dynamic "Write id.vi"("error in (no error)"=w2473, "id"=w2483, "Server in"=w2476) -> ("error out"=w2472:errorcluster, "Server out"=w2475:refnum<class "TCS.lvclass">)  [unwired: 7 in]
        n1445 = call-dynamic "Initialize.vi"("error in (no error)"=w2472, "TCS in"=w2475) -> ("error out"=w2470:errorcluster, "TCS out"=w2471:refnum<class "TCS.lvclass">)  [unwired: 8 in]
        n1446 = call-dynamic "Write TCS.lvclass.vi"("error in (no error)"=w2470, "TCS.lvclass"=w2471, "S4GUI in"=w2478) -> ("error out"=w2467:errorcluster, "S4GUI out"=w2468:refnum<class "S4GUI.lvclass">)  [unwired: 7 in]
      }
      event "enter password": Value Change {
        n1447 = event-data() -> ("NewVal"=w2484:bool)  [unwired: 1 in]
        n1448 = case shown="True" w2484 {
          tunnel: [w2490 w2492] -> w2488
          tunnel: [w2489 w2491] -> w2487
          tunnel: w2486 -> [w2490 w2505]
          tunnel: w2485 -> [w2489 w2504]
          frame False {
          }
          frame True {
            # "Verifica senha de configuração de CCD do Administrador"
            n1449 = Equal?(x="password", y="camerasetup") -> (x = y?=w2502:bool)
            n1450 = call-dynamic "Write mode Adm.vi"("error in (no error)"=w2504, "mode Adm"=w2502, "S4GUI in"=w2505) -> ("error out"=w2493:errorcluster, "S4GUI out"=w2494:refnum<class "S4GUI.lvclass">)  [unwired: 7 in]
